vi "UI_initialize.vi"(9 "本VI":refnum<vi>, 10 "簇":T1) -> ()   [LabVIEW 2018, in "UI.lvlib"]
uses:
  UI.lvlib
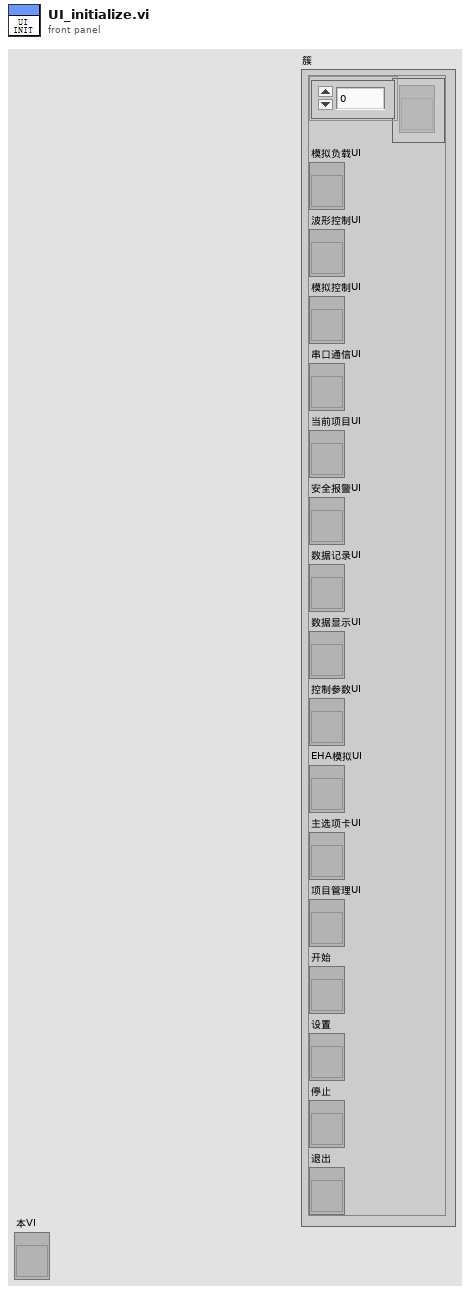
[diagram p1: front panel]
types:
  T1 = typedef "引用簇.ctl" = cluster{"数组":refnum<vi>[], "模拟负载UI":refnum<vi>, "波形控制UI":refnum<vi>, "模拟控制UI":refnum<vi>, "串口通信UI":refnum<vi>, "当前项目UI":refnum<vi>, "安全报警UI":refnum<vi>, "数据记录UI":refnum<vi>, "数据显示UI":refnum<vi>, "控制参数UI":refnum<vi>, "EHA模拟UI":refnum<vi>, "主选项卡UI":refnum<vi>, "项目管理UI":refnum<vi>, "开始":refnum<vi>, "设置":refnum<vi>, "停止":refnum<vi>, "退出":refnum<vi>}
  T2 = typedef "主选项卡枚举常量.ctl" = enum32{"开始页", "当前项目配置", "串口通信配置", "控制参数配置", "EHA模拟配置", "模拟控制配置", "模拟负载配置", "安全报警配置", "数据显示配置", "数据记录配置", "波形输出1", "波形输出2", "波形输出3", "波形输出4", "波形输出5", "波形输出6"}
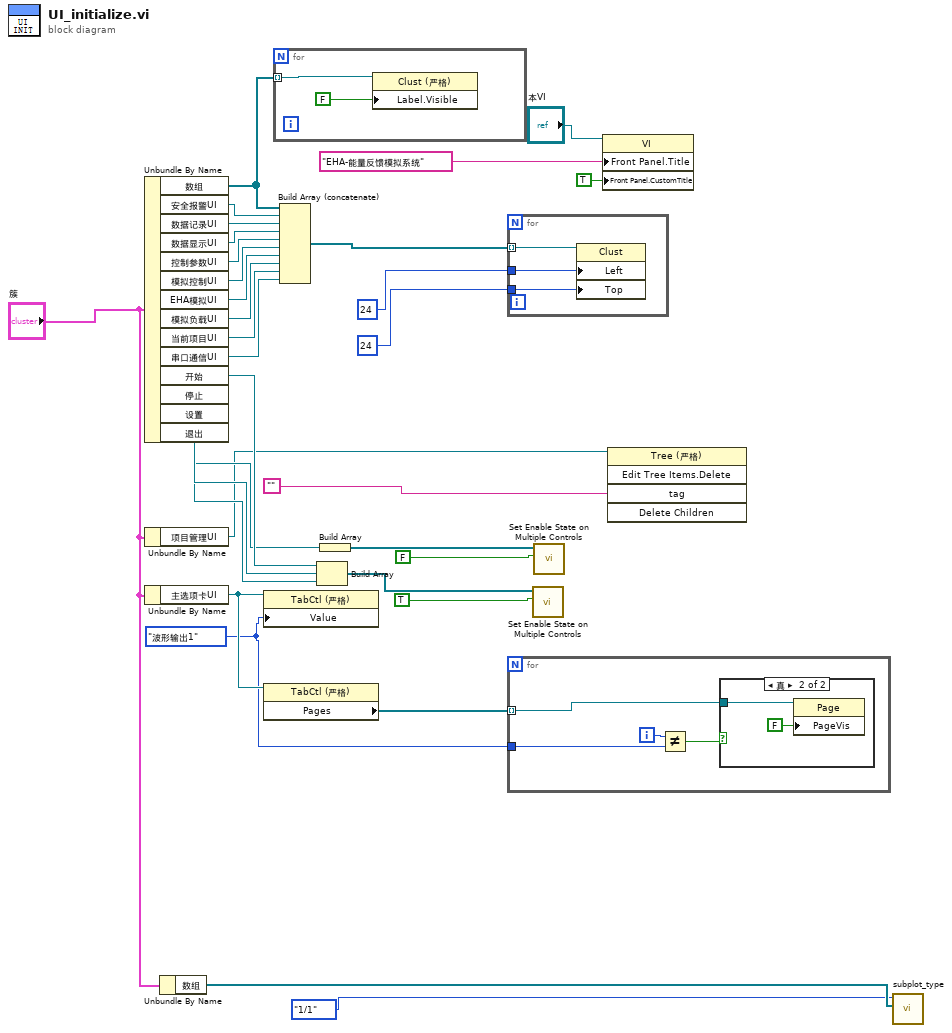
[diagram p0: block diagram]
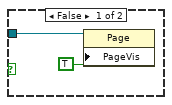
[diagram p2: hidden frame]
diagram:
  w3 = 主选项卡枚举常量."波形输出1" ("值")
  n1 = Unbundle By Name("簇") -> ("数组"=w2:refnum<vi>[], "安全报警UI"=w24:refnum<vi>, "数据记录UI"=w32:refnum<vi>, "数据显示UI"=w31:refnum<vi>, "控制参数UI"=w30:refnum<vi>, "模拟控制UI"=w29:refnum<vi>, "EHA模拟UI"=w28:refnum<vi>, "模拟负载UI"=w27:refnum<vi>, "当前项目UI"=w26:refnum<vi>, "串口通信UI"=w25:refnum<vi>, "开始"=w20:refnum<vi>, "停止"=w13:refnum<vi>, "设置"=w19:refnum<vi>, "退出"=w18:refnum<vi>)
  n2 = Unbundle By Name("簇") -> ("项目管理UI"=w8:refnum<vi>)
  n3 = Unbundle By Name("簇") -> ("主选项卡UI"=w6:refnum<vi>)
  n4 = Unbundle By Name("簇") -> ("数组"=w5:refnum<vi>[])
  n5 = property class="TabCtl (严格)"(reference=w6, "Value"=w3) -> ()  [unwired: 1 in, 2 out]
  n6 = property class="TabCtl (严格)"(reference=w6) -> ("Pages"=w7:refnum<vi>[])  [unwired: 1 in, 2 out]
  n7 = for {
    tunnel: w2 -> [w34] mode=indexing
    n8 = property class="Clust (严格)"(reference=w34, "Label.Visible"=FALSE ("标签.可见")) -> ()  [unwired: 1 in, 2 out]
  }
  n9 = Build Array (concatenate)(w2, w24, w32, w31, w30, w29, w28, w27, w26, w25) -> (w23:refnum<vi>[])
  n10 = Build Array(w20, w19, w18) -> (w17:refnum<vi>[])
  n11 = Build Array(w13) -> (w15:refnum<vi>[])
  n12 = for {
    tunnel: w23 -> [w37] mode=indexing
    tunnel: 24 ("位置:居左") -> [w36]
    tunnel: 24 ("位置:居左") -> [w35]
    n13 = property class="Clust"(reference=w37, "Left"=w36, "Top"=w35) -> ()  [unwired: 1 in, 2 out]
  }
  n14 = for {
    tunnel: w7 -> [w41] mode=indexing
    tunnel: w3 -> [w38]
    i -> [w39]
    n15 = Not Equal?(x=w39, y=w38) -> (x != y?=w40:bool)
    n16 = case shown="真" w40 {
      tunnel: w41 -> [w42 w45]
      frame False {
        n17 = property class="Page"(reference=w42, "PageVis"=TRUE ("选项卡可见")) -> ()  [unwired: 1 in, 2 out]
      }
      frame True {
        n18 = property class="Page"(reference=w45, "PageVis"=FALSE ("选项卡可见")) -> ()  [unwired: 1 in, 2 out]
      }
    }
  }
  n19 = call "Set Enable State on Multiple Controls.vi"("启用？"=TRUE, "控件"=w17) -> ()  [unwired: 10 in]
  n20 = call "Set Enable State on Multiple Controls.vi"("启用？"=FALSE, "控件"=w15) -> ()  [unwired: 10 in]
  n21 = property class="VI"(reference="本VI", "Front Panel.Title"="EHA-能量反馈模拟系统", "Front Panel.CustomTitle"=TRUE ("前面板窗口:自定义标题")) -> ()  [unwired: 1 in, 2 out]
  n22 = invoke class="Tree (严格)" method="Edit Tree Items.Delete"(reference=w8, "tag"="") -> ()  [unwired: 3 in, 5 out]
  n23 = call "subplot_type.vi"("数组"=w5, "枚举"=enum16{"1", "11", "1/1", "12", "1/2", "2/2"}."1/1") -> ()  [unwired: 10 in]
